vi "WPI_CAN_GetStatus.vi"(8 "error in (no error)":errorcluster) -> (0 "error out":errorcluster, 1 "Transmit Error Count":u32, 2 "Receive Error Count":u32, 3 "Percent Bus Utilization":sgl, 4 "Bus Off Count":u32, 6 "Transmit FIFO Full Count":u32)   [LabVIEW 2017]
doc: "This is the low-level CAN status VI. It may be used to monitor the health of the CAN bus.\n\n<b>Percent Bus Utilization</b> is an estimate of the amount of potential bandwidth that was used in a recent time-frame.\n\n<b>Receive Error Count</b> and <b>Transmit Error Count</b> report the status of the CAN controller's REC and TEC registers.\n\n<b>Bus Off Count</b> is the number of times that the CAN controller reported a \"Bus Off\" state and was reset.\n\n<b>Transmit FIFO Full Count</b> is the number of times that the transmit FIFO was reported as full after being drained."
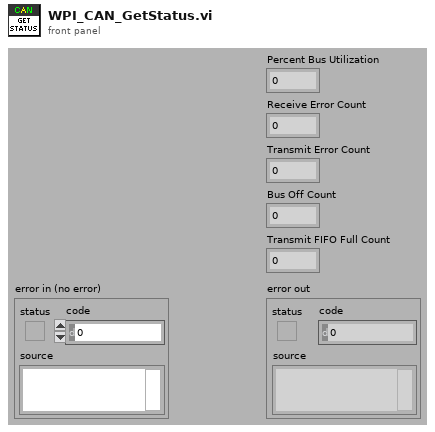
[diagram p1: front panel]
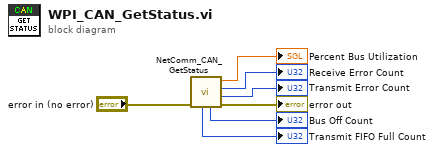
[diagram p0: block diagram]
diagram:
  n1 = call <vilib>:"NetComm_CAN_GetStatus.vi"("error in (no error)"="error in (no error)") -> ("error out"=→"error out":errorcluster, "Transmit Error Count"=→"Transmit Error Count":u32, "Receive Error Count"=→"Receive Error Count":u32, "Percent Bus Utilization"=→"Percent Bus Utilization":sgl, "Bus Off Count"=→"Bus Off Count":u32, "Transmit FIFO Full Count"=→"Transmit FIFO Full Count":u32)  [unwired: 5 in]
